vi "MVE Read Setting.vi"(11 "key":string) -> (2 "value":string, 3 "Success":bool)   [LabVIEW 2016]
uses:
  <resource>/dialog/lvconfig.llb/LV Config Read String.vi
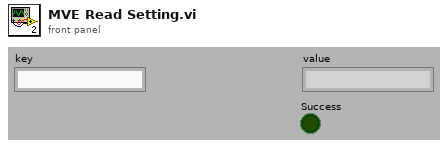
[diagram p1: front panel]
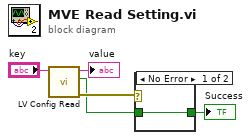
[diagram p0: block diagram]
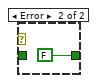
[diagram p2: hidden frame]
diagram:
  n1 = call-poly <resource>:"LV Config Read.vi"("key"="key") -> ("error out"=w3:errorcluster, "found?"=w2:bool, "value"=→"value":string)  [unwired: 4 in]
  n2 = case shown="No Error" w3 {
    tunnel: w2 -> [w6 _]
    tunnel: [w6 FALSE ("found?")] -> w1
    frame No Error {
    }
    frame Error {
    }
  }
  "Success" <- w1
